vi "VFH 루프.vi"() -> ()   [LabVIEW 2016]
uses:
  <vilib>/Platform/TimedLoop/XDataNode/wakeup.ctl
  <vilib>/Platform/TimedLoop/XDataNode/XDNodeRunTimeDep.lvlib
  <vilib>/Platform/TimedLoop/XDataNode/nitl_modes.ctl
  <vilib>/Platform/TimedLoop/XDataNode/timing_clust.ctl
  <vilib>/Platform/TimedLoop/XDataNode/XDataNode.xnode
panel:
  in  "obstacle clearance distance":dbl=0.420745
  out "mask":bool[](array[boolean])
  out "histogram":dbl[](array[numeric])
  in  "error in":errorcluster
  out "Distance":dbl[](array[numeric])
  out "Angle":dbl[](array[numeric])
  in  "Target Angle":dbl
  in  "출력 클러스터":T1
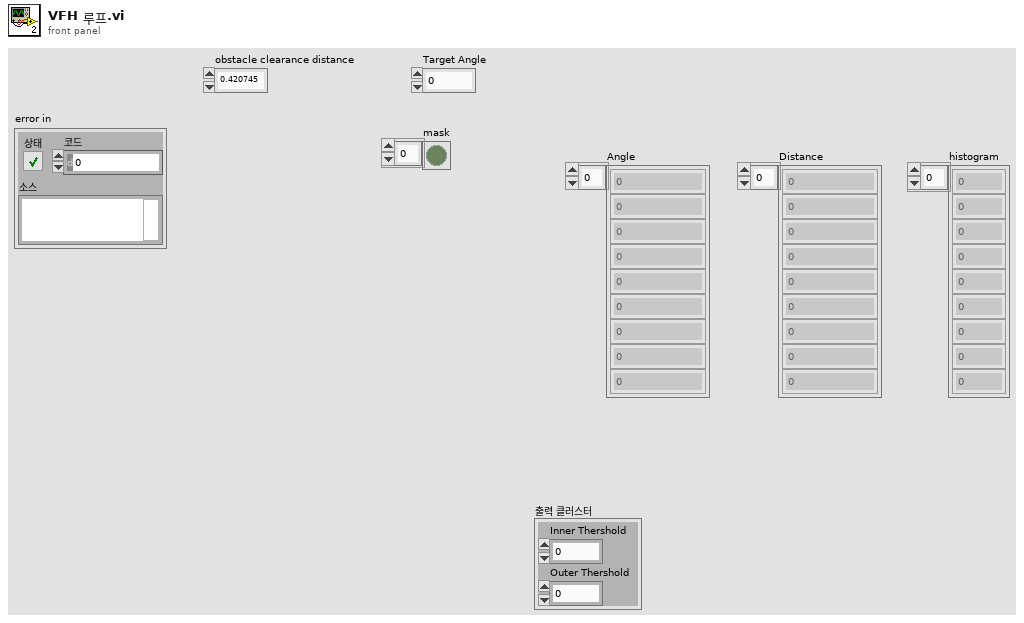
[diagram p1: front panel]
types:
  T1 = cluster{"Inner Thershold":dbl, "Outer Thershold":dbl}
  T2 = typedef "XDNodeRunTimeDep.lvlib/timing_clust.ctl" = cluster{"Expected End [f-1]":u64, "Actual End [f-1]":u64, "Finished Late? [f-1]":bool, "Expected End [i-1]":u64, "Actual End [i-1]":u64, "Finished Late? [i-1]":bool, "Expected Start [i]":u64, "Actual Start [i]":u64, "Expected Start [f]":u64, "Actual Start [f]":u64, "Source Name":string, "Structure Name":string, "Period":i64, "Deadline":i64, "Offset":i64, "Start":i64, "Priority":i32, "Timeout":i32, "Mode":T3, "Wakeup Reason":T4, "Error":errorcluster, "Source Type":string, "Secondary Source Type":string, "Global End Time":u64, "Global Start Time":u64, "Frame Duration":u64, "Iteration Duration":u64, "Assigned CPU":i32, "I/O Scan Engine Mode":u32}
  T3 = typedef "XDNodeRunTimeDep.lvlib/nitl_modes.ctl" = enum32{"No Change", "Process missed periods, maintain original phase", "Discard missed periods, maintain original phase", "Process missed periods, ignore original phase", "Discard missed periods, ignore original phase"}
  T4 = typedef "XDNodeRunTimeDep.lvlib/wakeup.ctl" = enum32{"Normal", "Aborted", "Asynchronous wakeup", "Timing source error", "Timed loop error", "Timeout"}
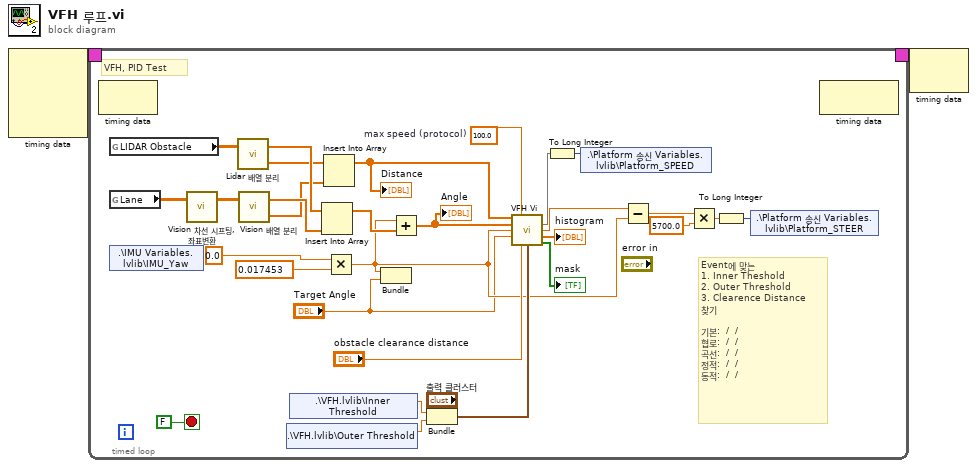
[diagram p0: block diagram]
diagram:
  n1 = node-c288() -> (w2:T2)  [unwired: 4 in]
  n2 = timed-loop {
    timing: w2 -> [_]
    timing-out: [_] -> w1
    stop <- FALSE stop-if-true
    w6 = 100.0  # max speed (protocol)
    # "Event에 맞는\n1. Inner Theshold\n2. Outer Threshold\n3. Clearence Distance\n찾기\n\n기본:  /  /  \n협로:  /  /\n곡선:  /  /\n정적:  /  /\n동적:  /  /"
    # "VFH, PID Test"
    n3 = node-c288() -> ()  [unwired: 1 in, 1 out]
    n4 = global read "[GV]_Lidar Obstacle.vi" "LIDAR Obstacle"() -> (w26:dbl[][])
    n5 = global read "[GV]_Vision Lane.vi" "Lane"() -> (w5:dbl[][])
    n6 = shared-variable ".\\IMU Variables.lvlib\\IMU_Yaw"() -> ()  [unwired: 1 in, 2 out]
    n7 = call "Vision 차선 시프팅, 좌표변환.vi"("VIsion"=w5) -> ("Vision"=w4:dbl[][])  [unwired: 2 in, 2 out]
    n8 = call "Lidar 배열 분리.vi"("행렬"=w26) -> ("Lidar Distance (m)"=w22:dbl[], "Lidar Angle (rad)"=w24:dbl[])  [unwired: 1 in]
    n9 = call "Vision 배열 분리.vi"("Vision Data"=w4) -> ("Vision Distance (m)"=w23:dbl[], "Vision Angle (rad)"=w25:dbl[])  [unwired: 1 in]
    n10 = shared-variable ".\\VFH.lvlib\\Outer Threshold"() -> (w3:dbl)  [unwired: 1 in, 1 out]
    n11 = shared-variable ".\\VFH.lvlib\\Inner Threshold"() -> (w19:dbl)  [unwired: 1 in, 1 out]
    n12 = Insert Into Array(array=w24, new element=w25) -> (w21:dbl[])  [unwired: 1 in]
    n13 = Insert Into Array(array=w22, new element=w23) -> (w14:dbl[])  [unwired: 1 in]
    "Distance" <- w14
    n14 = Multiply(x=0.0, y=0.017453 ("GPS_Longitude 2")) -> (x*y=w12:dbl)
    n15 = Bundle(w12, "Target Angle"="Target Angle") -> ()  [unwired: 1 in, 1 out]
    n16 = Add(x=w12, y=w21) -> (x+y=w13:dbl[])
    "Angle" <- w13
    n17 = Bundle(cluster="출력 클러스터", "Inner Thershold"=w19, "Outer Thershold"=w3) -> (w18:T1)
    n18 = call "VFH Vi.vi"("LIDAR & Vision magn. (m)"=w14, 1:w6, "LIDAR & Vision angle (rad)"=w13, "current heading (rad)"=w12, "target heading (rad)"="Target Angle", "obstacle clearance (m)"="obstacle clearance distance", "thresholds"=w18) -> (6:w9, "command heading (rad)"=w11:dbl, "histogram out"=→"histogram":dbl[], "mask out"=→"mask":bool[])  [unwired: 5 in]
    n19 = To Long Integer(number=w9) -> (32bit integer=w8:i32)
    n20 = shared-variable ".\\Platform 송신 Variables.lvlib\\Platform_SPEED"(w8) -> ()  [unwired: 1 in, 1 out]
    n21 = Subtract(x=w11, y=w12) -> (x-y=w27:dbl)
    n22 = Multiply(x=w27, y=5700.0) -> (x*y=w30:dbl)
    n23 = To Long Integer(number=w30) -> (32bit integer=w29:i32)
    n24 = shared-variable ".\\Platform 송신 Variables.lvlib\\Platform_STEER"(w29) -> ()  [unwired: 1 in, 1 out]
    n25 = node-c288() -> ()  [unwired: 1 in, 1 out]
  }
  n26 = node-c288(w1) -> ()  [unwired: 1 out]
